vi "3-lorentzian-heat-response -- V3.vi"(7 "action":T1, 8 "m1m2m3 IN":dbl[](array[numeric])=[-0.0007412078466363201, -0.0004027798896083045, -0.019859061457473383, -0.00809909374498405, -0.08771864860021968, -0.6888815311338856], 10 "parameters IN":dbl[](array[numeric])=[-0.0007412078466363201, -0.0004027798896083045, -0.019859061457473383, -0.00809909374498405, -0.08771864860021968, -0.6888815311338856], 11 "omega IN (rad/sec)":dbl=0.1 format="%#_10f") -> (0 "m1m2m3 OUT":dbl[](array[numeric])=[-0.0007412078466363201, -0.0004027798896083045, -0.019859061457473383, -0.00809909374498405, -0.08771864860021968, -0.6888815311338856], 1 "Romega":cdb=0.1+0.0i format="%#_10f", 2 "parameters OUT":dbl[](array[numeric])=[-0.0007412078466363201, -0.0004027798896083045, -0.019859061457473383, -0.00809909374498405, -0.08771864860021968, -0.6888815311338856], 3 "omega OUT(rad/sec)":dbl=0.1 format="%#_10f", 4 "String out":string)   [LabVIEW 2020]
uses:
  3-lorentzian-heat-response action.ctl
  142dd4c5-f9ed-c64b-bc14-a88e3e2c450a.vi
  <vilib>/Analysis/polynomials.llb/Multiply Polynomials (DBL).vi
  <vilib>/Analysis/polynomials.llb/Polynomial Roots (DBL).vi
  <vilib>/Comparison/Less/Less Functor/Less Functor.lvclass
  <vilib>/Analysis/NI_AALPro.lvlib
panel:
  out "m1":dbl=0.1 format="%#_10f"
  out "m2":dbl=0.1 format="%#_10f"
  out "m3":dbl=0.1 format="%#_10f"
  in  "m1 IN":dbl=0.1 format="%#_10f"
  in  "m2 IN":dbl=0.1 format="%#_10f"
  in  "m3 IN":dbl=0.1 format="%#_10f"
  in  "kappa0":dbl(slide)=0.000285 min=0.0 max=0.3 step=1e-06 scale=0.01..10.0 scale format="%#_3p"
  in  "tauC":dbl(slide)=0.000285 min=0.0 max=0.3 step=1e-06 scale=0.01..10.0 scale format="%#_3p"
  in  "tauN":dbl(slide)=0.000285 min=0.0 max=0.3 step=1e-06 scale=0.01..10.0 scale format="%#_3p"
  in  "tauS":dbl(slide)=0.000285 min=0.0 max=0.3 step=1e-06 scale=0.01..10.0 scale format="%#_3p"
  in  "T1":dbl(slide)=0.000285 min=0.0 max=0.3 step=1e-06 scale=0.01..10.0 scale format="%#_3p"
  in  "zeta":dbl(slide)=0.000285 min=0.0 max=0.3 step=1e-06 scale=0.01..10.0 scale format="%#_3p"
  in  "what":cluster{"derivative":T1, "scaling":dbl}[](array[cluster])=[{"derivative"=enum."dζ", "scaling"=1.0}, {"derivative"=enum."dT1", "scaling"=1.0}, {"derivative"=enum."dτS", "scaling"=1.0}, {"derivative"=enum."dτN", "scaling"=1.0}, {"derivative"=enum."dτC", "scaling"=1.0}, {"derivative"=enum."dκ0", "scaling"=0.0}]
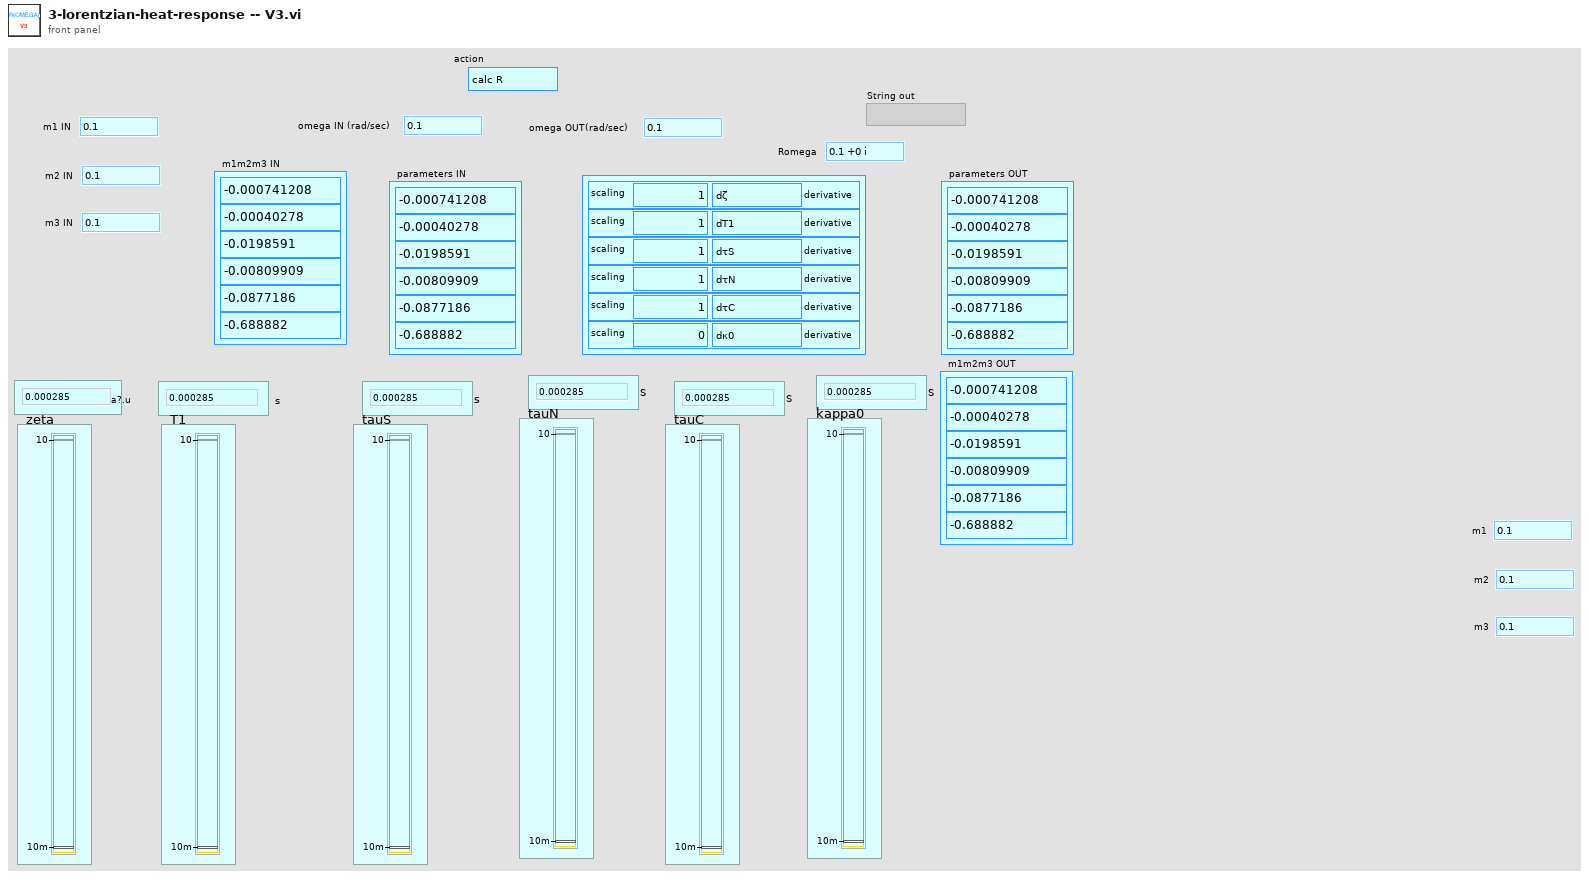
[diagram p1: front panel]
types:
  T1 = typedef "3-lorentzian-heat-response action.ctl" = enum16{"calc R", "create string", "calc m1m2m3", "dζ", "dT1", "dτS", "dτN", "dτC", "d-all", "dκ0", "T(K)", "m1", "m2", "m3", "parse string", "θ (deg)", "B (T)"}
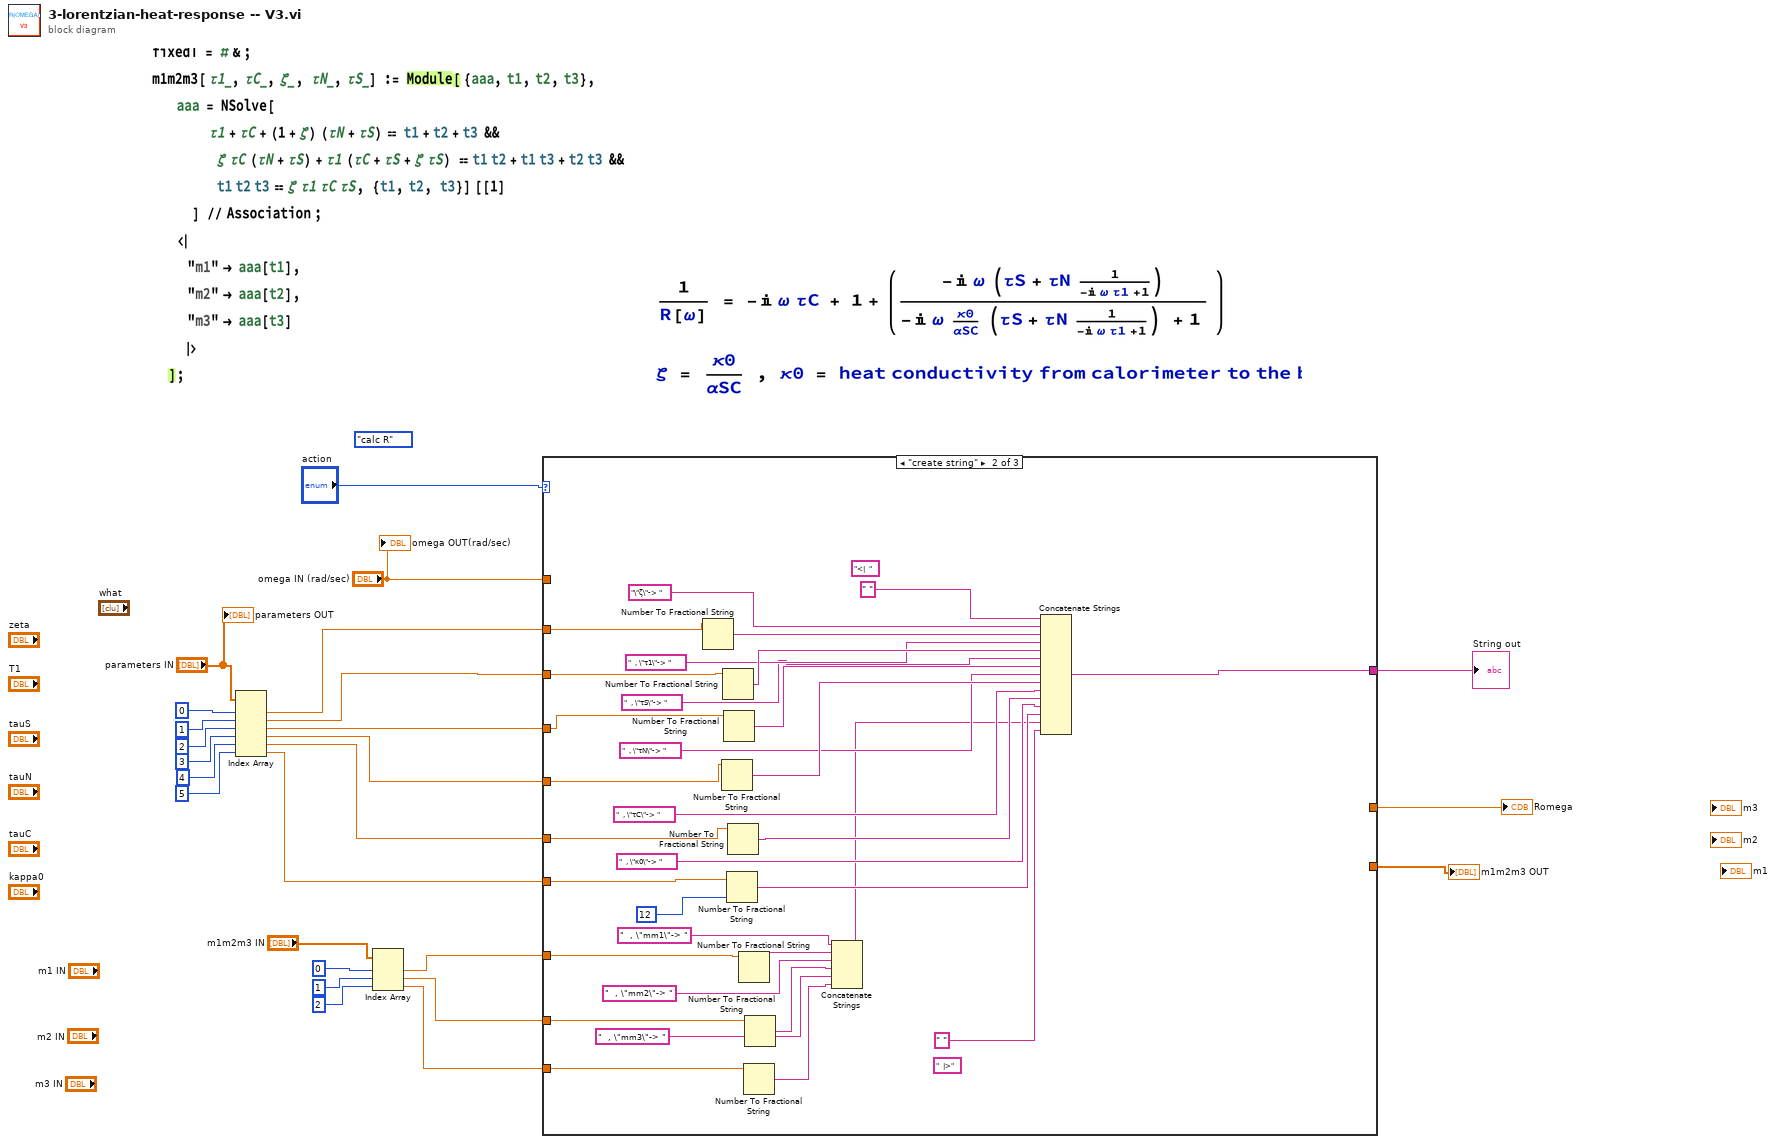
[diagram p0: block diagram]
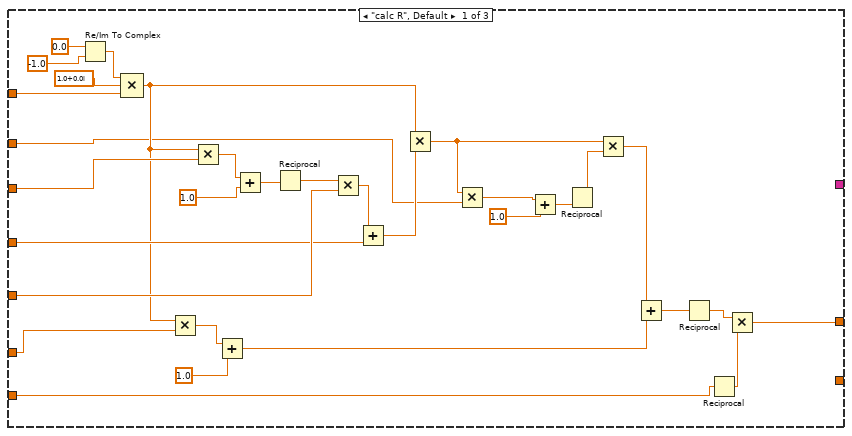
[diagram p2: hidden frame]
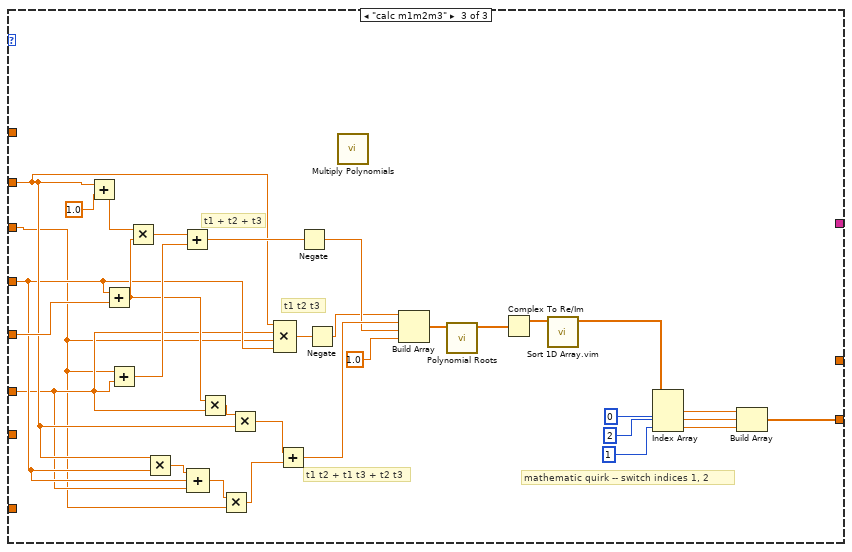
[diagram p3: hidden frame]
diagram:
  (unwired) 3-lorentzian-heat-response_action."calc R" ("action")
  n1 = Index Array(array="parameters IN", index #1=0 ("index"), index #2=1 ("index"), index #3=2 ("index"), index #4=3 ("index"), index #5=4 ("index"), index #6=5 ("index")) -> (element #1=w16:dbl, element #2=w15:dbl, element #3=w14:dbl, element #4=w13:dbl, element #5=w12:dbl, element #6=w11:dbl)
  n2 = Index Array(array="m1m2m3 IN", index #1=0 ("index"), index #2=1 ("index"), index #3=2 ("index")) -> (element #1=w6:dbl, element #2=w5:dbl, element #3=w4:dbl)
  n3 = case shown="\"create string\"" "action" {
    tunnel: w12 -> [w42 w86 w106]
    tunnel: "omega IN (rad/sec)" -> [w45 _ _]
    tunnel: w15 -> [w44 w87 w104]
    tunnel: w13 -> [w50 w79 w119]
    tunnel: w14 -> [w48 w80 w107]
    tunnel: w16 -> [w38 w88 w109]
    tunnel: [w26 _ _] -> w24
    tunnel: w11 -> [w29 w85 _]
    tunnel: [_ w70 _] -> w23
    tunnel: w6 -> [_ w68 _]
    tunnel: w5 -> [_ w67 _]
    tunnel: w4 -> [_ w66 _]
    tunnel: [_ _ w89] -> w1
    frame "calc R", Default {
      n4 = Re/Im To Complex(1:-1.0 ("y"), 2:0.0 ("x")) -> (0:w46:cdb)
      n5 = Compound Arithmetic op=MULTIPLY(w46, cdb 1.0+0.0i ("value"), w45) -> (w40:cdb)
      n6 = Multiply(x=w40, y=w42) -> (x*y=w41:cdb)
      n7 = Multiply(x=w40, y=w44) -> (x*y=w43:cdb)
      n8 = Add(x=w41, y=1.0) -> (x+y=w32:cdb)
      n9 = Add(x=w43, y=1.0) -> (x+y=w52:cdb)
      n10 = Reciprocal(x=w52) -> (1/x=w51:cdb)
      n11 = Multiply(x=w51, y=w50) -> (x*y=w49:cdb)
      n12 = Add(x=w49, y=w48) -> (x+y=w39:cdb)
      n13 = Multiply(x=w40, y=w39) -> (x*y=w34:cdb)
      n14 = Multiply(x=w34, y=w38) -> (x*y=w36:cdb)
      n15 = Add(x=w36, y=1.0) -> (x+y=w35:cdb)
      n16 = Reciprocal(x=w35) -> (1/x=w33:cdb)
      n17 = Multiply(x=w34, y=w33) -> (x*y=w31:cdb)
      n18 = Add(x=w31, y=w32) -> (x+y=w30:cdb)
      n19 = Reciprocal(x=w30) -> (1/x=w28:cdb)
      n20 = Reciprocal(x=w29) -> (1/x=w27:dbl)
      n21 = Multiply(x=w28, y=w27) -> (x*y=w26:cdb)
    }
    frame "create string" {
      (unwired) "<|  "
      (unwired) "  |>"
      n22 = Number To Fractional String(number=w88) -> (F-format string=w84:string)  [unwired: 3 in]
      n23 = Number To Fractional String(number=w79) -> (F-format string=w81:string)  [unwired: 3 in]
      n24 = Number To Fractional String(number=w87) -> (F-format string=w83:string)  [unwired: 3 in]
      n25 = Number To Fractional String(number=w80) -> (F-format string=w82:string)  [unwired: 3 in]
      n26 = Number To Fractional String(number=w85, precision (6)=i16 12 ("width (-)")) -> (F-format string=w71:string)  [unwired: 2 in]
      n27 = Number To Fractional String(number=w86) -> (F-format string=w73:string)  [unwired: 3 in]
      n28 = Number To Fractional String(number=w68) -> (F-format string=w64:string)  [unwired: 3 in]
      n29 = Number To Fractional String(number=w66) -> (F-format string=w60:string)  [unwired: 3 in]
      n30 = Number To Fractional String(number=w67) -> (F-format string=w62:string)  [unwired: 3 in]
      n31 = Concatenate Strings("  , \"mm1\"-> ", w64, "  , \"mm2\"-> ", w62, "  , \"mm3\"-> ", w60) -> (w59:string)
      n32 = Concatenate Strings(" ", "\"ζ\"-> ", w84, "  , \"τ1\"-> ", w83, "  , \"τS\"-> ", w82, "  , \"τN\"-> ", w81, "  , \"τC\"-> ", w73, "  , \"κ0\"-> ", w71, w59, " ") -> (w70:string)
    }
    frame "calc m1m2m3" {
      # "mathematic quirk -- switch indices 1, 2"
      # "t1 t2 + t1 t3 + t2 t3"
      # "t1 + t2 + t3"
      # "t1 t2 t3"
      n33 = Add(x=w109, y=1.0) -> (x+y=w118:dbl)
      n34 = Add(x=w107, y=w119) -> (x+y=w111:dbl)
      n35 = Add(x=w104, y=w106) -> (x+y=w116:dbl)
      n36 = Multiply(x=w118, y=w111) -> (x*y=w117:dbl)
      n37 = Multiply(x=w109, y=w107) -> (x*y=w108:dbl)
      n38 = Add(x=w117, y=w116) -> (x+y=w112:dbl)
      n39 = Compound Arithmetic op=ADD(w108, w107, w106) -> (w105:dbl)
      n40 = Multiply(x=w111, y=w106) -> (x*y=w110:dbl)
      n41 = Multiply(x=w105, y=w104) -> (x*y=w102:dbl)
      n42 = Multiply(x=w110, y=w109) -> (x*y=w103:dbl)
      n43 = Compound Arithmetic op=MULTIPLY(w109, w106, w104, w107) -> (w115:dbl)
      n44 = Add(x=w103, y=w102) -> (x+y=w101:dbl)
      n45 = Negate(x=w112) -> (-x=w94:dbl)
      n46 = Negate(x=w115) -> (-x=w93:dbl)
      n47 = call-poly <vilib>:"Multiply Polynomials.vi"() -> ()  [unwired: 10 in, 2 out]
      n48 = Build Array(w93, w101, w94, 1.0 ("element")) -> (w113:dbl[])
      n49 = call-poly <vilib>:"Polynomial Roots.vi"("P(x)"=w113) -> ("Roots"=w96:cdb[])  [unwired: 9 in, 1 out]
      n50 = Complex To Re/Im(x + iy=w96) -> (x=w95:dbl[])  [unwired: 1 out]
      n51 = call "Sort 1D Array.vim"("unsorted array"=w95) -> ("sorted array"=w97:dbl[])  [unwired: 10 in]
      n52 = Index Array(array=w97, index #1=0 ("index"), index #2=2 ("index"), index #3=1 ("index")) -> (element #1=w92:dbl, element #2=w91:dbl, element #3=w90:dbl)
      n53 = Build Array(w92, w91, w90) -> (w89:dbl[])
    }
  }
  "Romega" <- w24
  "String out" <- w23
  "m1m2m3 OUT" <- w1
  "parameters OUT" <- "parameters IN"
  "omega OUT(rad/sec)" <- "omega IN (rad/sec)"
